vi "SQL数据read.vi"(0 "database":string(combo), 1 "condition":string, 2 "Password":string="783523103", 5 "table输入":string(combo), 7 "枚举":enum16{"DBTOOL", "SQLquery"}(ring), 9 "columns":string[](array[string]), 11 "error in (no error)":errorcluster, 12 "SQL query":string) -> (4 "data":string[][](table), 6 "子数组":string[](array[string]), 15 "error out":errorcluster)   [LabVIEW 2016]
uses:
  <vilib>/Utility/sysdir.llb/System Directory Type.ctl
  <vilib>/addons/database/Connection.llb/DB Tools Open Connec (String).vi
  <vilib>/addons/database/Connection.llb/Conn Execute.vi
  <vilib>/addons/database/Recordset.llb/Rec Fetch Recordset Data (R).vi
  <vilib>/addons/database/Recordset.llb/Rec Destroy - Connection.vi
  <vilib>/addons/database/_DB Variant To Data/Database Variant To Data.xnode
  <vilib>/addons/database/NI_Database_API.lvlib
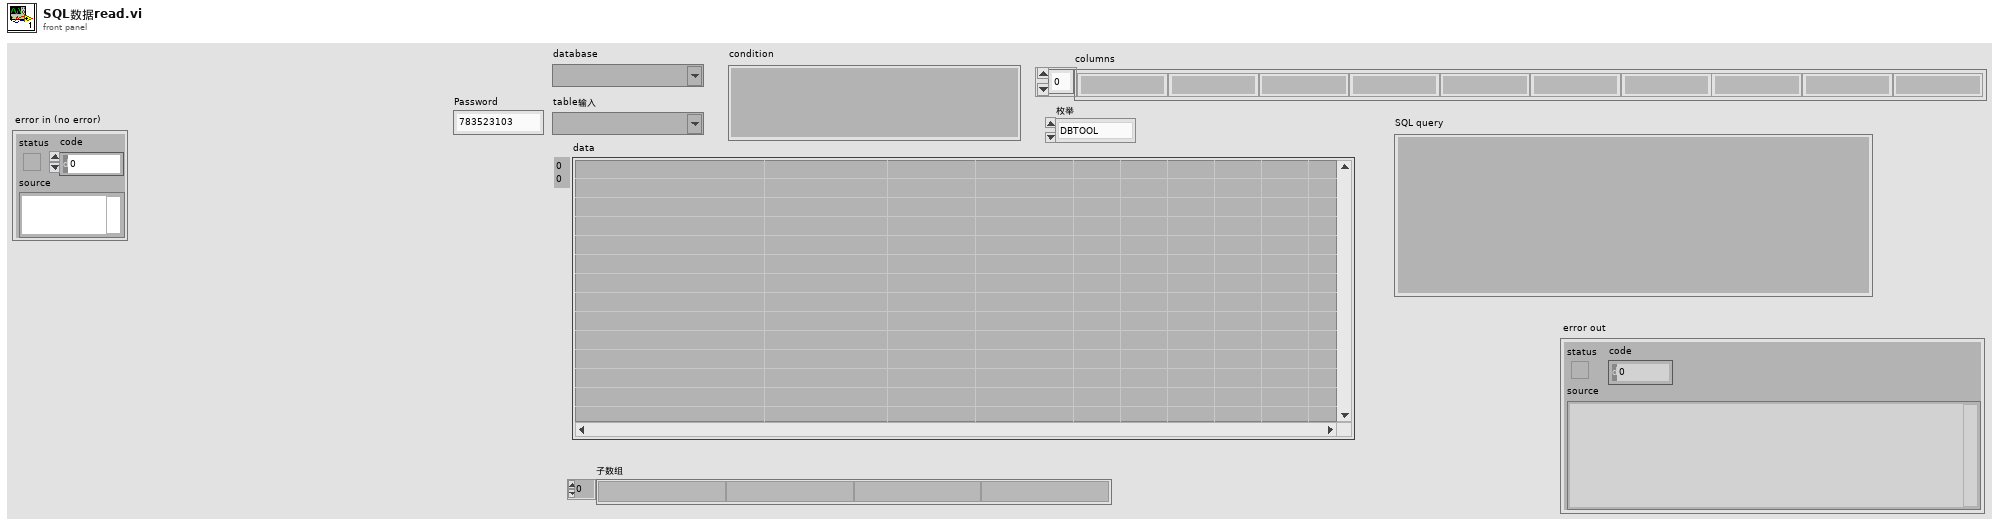
[diagram p1: front panel]
types:
  T1 = typedef "System Directory Type.ctl" = i32
  T2 = typedef "NI_Database_API.lvlib/Conn ObjectReference.ctl" = refnum<k1>
  T3 = typedef "NI_Database_API.lvlib/Rec ObjectReference.ctl" = refnum<k1>
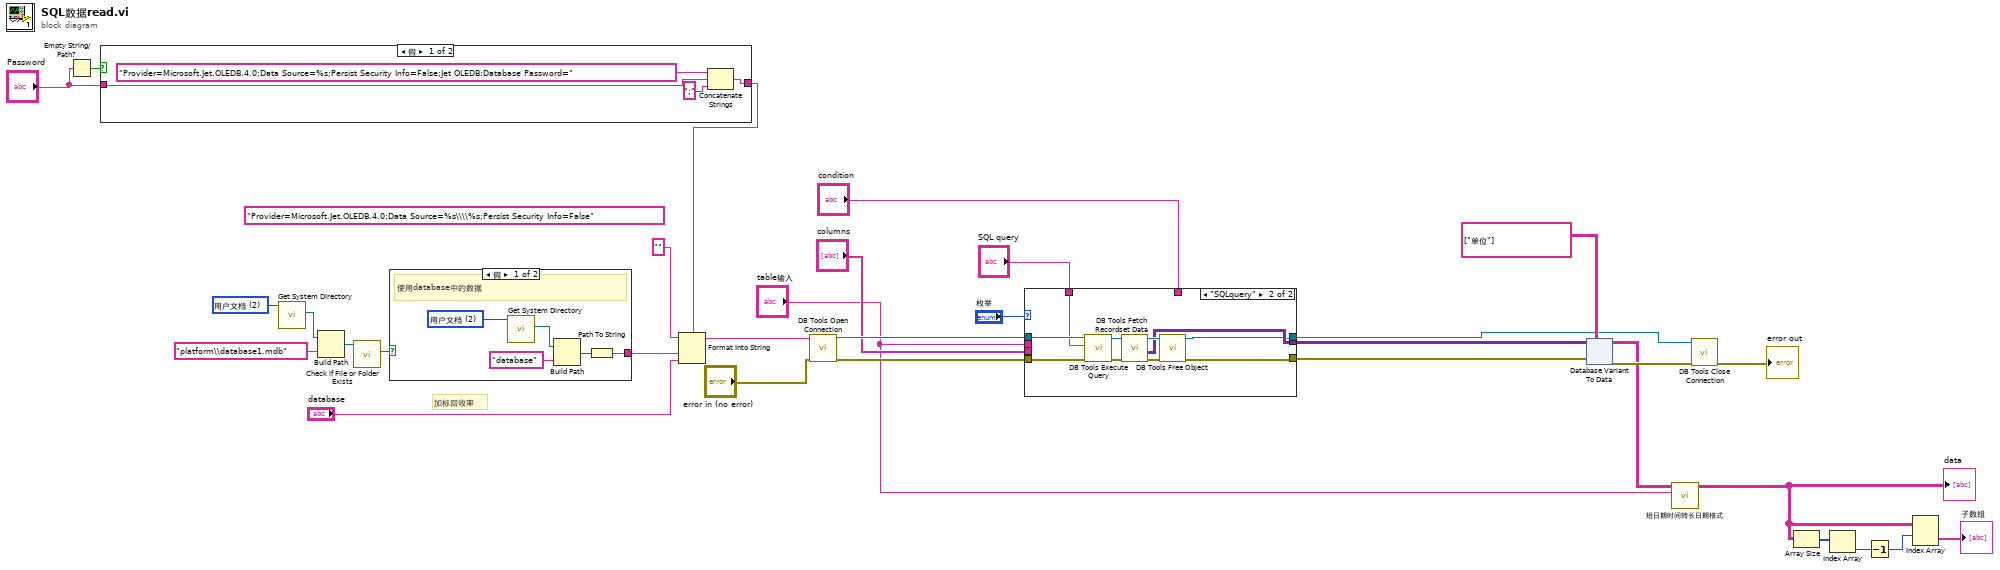
[diagram p0: block diagram]
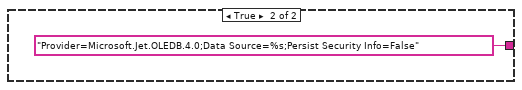
[diagram p2: hidden frame]
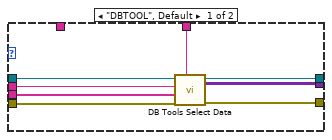
[diagram p3: hidden frame]
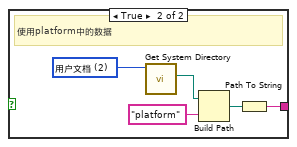
[diagram p4: hidden frame]
diagram:
  w29 = T1 2 items=["用户目录"=0, "用户桌面"=1, "用户文档"=2, "用户应用程序数据"=3, "用户设置"=4, "用户临时目录"=5, "公共文档"=6, "公共应用程序数据"=7, "公共设置"=8, "公共缓存"=13, "系统核心库"=9, "系统安装库"=10, "应用程序文件"=11, "启动盘根目录"=12] ("system directory type")
  (unwired) "Provider=Microsoft.Jet.OLEDB.4.0;Data Source=%s\\\\%s;Persist Security Info=False" ("格式字符串")
  # "加标回收率"
  n1 = Empty String/Path?(string/path="Password") -> (empty?=w2:bool)
  n2 = case shown="假" w2 {
    tunnel: [w33 "Provider=Microsoft.Jet.OLEDB.4.0;Data Source=%s;Persist Security Info=False" ("格式字符串")] -> w1
    tunnel: "Password" -> [w36 _]
    frame False {
      n3 = Concatenate Strings("Provider=Microsoft.Jet.OLEDB.4.0;Data Source=%s;Persist Security Info=False;Jet OLEDB:Database Password=" ("格式字符串"), w36, ";" ("字符串")) -> (w33:string)
    }
    frame True {
    }
  }
  n4 = call <vilib>:"Get System Directory.vi"("system directory type"=w29) -> ("system directory"=w30:path)  [unwired: 10 in]
  n5 = Build Path(base path=w30, name or relative path="platform\\database1.mdb" ("condition")) -> (appended path=w28:path)
  n6 = call <vilib>:"Check if File or Folder Exists.vi"("path"=w28) -> ("file or folder exists?"=w26:bool)  [unwired: 8 in, 2 out]
  n7 = case shown="假" w26 {
    tunnel: [w38 w43] -> w25
    frame False {
      w41 = T1 2 items=["用户目录"=0, "用户桌面"=1, "用户文档"=2, "用户应用程序数据"=3, "用户设置"=4, "用户临时目录"=5, "公共文档"=6, "公共应用程序数据"=7, "公共设置"=8, "公共缓存"=13, "系统核心库"=9, "系统安装库"=10, "应用程序文件"=11, "启动盘根目录"=12] ("system directory type")
      # "使用database中的数据"
      n8 = call <vilib>:"Get System Directory.vi"("system directory type"=w41) -> ("system directory"=w40:path)  [unwired: 10 in]
      n9 = Build Path(base path=w40, name or relative path="database" ("condition")) -> (appended path=w42:path)
      n10 = Path To String(path=w42) -> (string=w38:string)
    }
    frame True {
      w47 = T1 2 items=["用户目录"=0, "用户桌面"=1, "用户文档"=2, "用户应用程序数据"=3, "用户设置"=4, "用户临时目录"=5, "公共文档"=6, "公共应用程序数据"=7, "公共设置"=8, "公共缓存"=13, "系统核心库"=9, "系统安装库"=10, "应用程序文件"=11, "启动盘根目录"=12] ("system directory type")
      # "使用platform中的数据"
      n11 = call <vilib>:"Get System Directory.vi"("system directory type"=w47) -> ("system directory"=w46:path)  [unwired: 10 in]
      n12 = Build Path(base path=w46, name or relative path="platform" ("condition")) -> (appended path=w44:path)
      n13 = Path To String(path=w44) -> (string=w43:string)
    }
  }
  n14 = Format Into String(format string=w1, initial string="" ("初始字符串"), w25, "database") -> (resulting string=w24:string)  [unwired: 1 in, 1 out]
  n15 = call-poly <vilib>:"DB Tools Open Connection.vi"("error in (no error)"="error in (no error)", "connection information"=w24) -> ("error out"=w21:errorcluster, "connection reference"=w22:T2)  [unwired: 6 in]
  n16 = case shown="\"SQLquery\"" "枚举" {
    tunnel: w22 -> [w55 w61]
    tunnel: w21 -> [w54 w59]
    tunnel: "columns" -> [w53 _]
    tunnel: "condition" -> [w52 _]
    tunnel: [w51 w56] -> w17
    tunnel: [w50 w58] -> w16
    tunnel: [w49 w57] -> w15
    tunnel: "table输入" -> [w48 _]
    tunnel: "SQL query" -> [_ w60]
    frame "DBTOOL", Default {
      n17 = call <vilib>:"DB Tools Select Data.vi"("condition"=w52, "error in (no error)"=w54, "columns"=w53, "table"=w48, "connection reference"=w55) -> ("error out"=w51:errorcluster, "data"=w50:variant[][], "connection reference out"=w49:T2)  [unwired: 1 in]
    }
    frame "SQLquery" {
      n18 = call-poly <vilib>:"DB Tools Execute Query.vi"("error in (no error)"=w59, "SQL query"=w60, "connection reference"=w61) -> ("error out"=w65:errorcluster, "recordset reference"=w63:T3)  [unwired: 5 in]
      n19 = call-poly <vilib>:"DB Tools Fetch Recordset Data.vi"("error in (no error)"=w65, "recordset reference"=w63) -> ("error out"=w62:errorcluster, "recordset data"=w58:variant[][], "recordset reference out"=w64:T3)  [unwired: 3 in]
      n20 = call-poly <vilib>:"DB Tools Free Object.vi"("error in (no error)"=w62, "recordset reference"=w64) -> ("error out"=w56:errorcluster, "connection reference"=w57:T2)  [unwired: 8 in]
    }
  }
  n21 = xnode "Database Variant To Data"("database variant"=w16, "error in (no error)"=w17, "type"=string[][] [["单位"]]) -> ("data"=w7:string[][], "error out"=w14:errorcluster)
  n22 = call "短日期时间转长日期格式.vi"("table输入"="table输入", "data"=w7) -> ("输出数组"=w6:string[][])  [unwired: 9 in]
  "data" <- w6
  n23 = call <vilib>:"DB Tools Close Connection.vi"("error in (no error)"=w14, "connection reference"=w15) -> ("error out"=→"error out":errorcluster)  [unwired: 5 in]
  n24 = Array Size(array=w6) -> (size(s)=w11:i32[])
  n25 = Index Array(array=w11) -> (element=w9:i32)  [unwired: 1 in]
  n26 = Decrement(x=w9) -> (x-1=w8:i32)
  n27 = Index Array(array=w6, index (row)=w8) -> (element=→"子数组":string[])  [unwired: 1 in]
